vi "Main.vi"() -> ()   [LabVIEW 2025]
doc: "This template is for the Queued Message Handler design pattern.\n\nThe Event Handling Loop generates messages based on user interface actions.\n\nThe Message Handling Loop processes messages generated by the Event Handling Loop, or by other messages. The messages are string values, so new messages can be added easily to the Message Cases case structure in the Message Handling Loop. Each message cluster can also provide an optional value for Message Data, which is a variant that can be converted to whatever message-specific data is required."
uses:
  support/Message Queue/Enqueue Message (Single).vi
  <vilib>/Utility/error.llb/Error Cluster From Error Code.vi
  <vilib>/ErrorRing/Error Ring.xnode
  support/Message Queue/Message Queue.lvlib
  support/User Event - Stop/User Event - Stop.lvlib
panel:
  out "Status":string
  out "Counter Status":bool
  in  "Speed: [Knob: 1-5]":i32(knob) scale=1.0..5.0
  in  "Pause":bool
  in  "Play":bool
  out "Counter":dbl
  in  "Exit":bool
  # "Counter"
  # "Use the Play, Pause, and Exit buttons to control the primary counting function.\n\nThe Play button initiates or resumes the counter.\nPause will temporarily halt the counter, allowing you to resume from the same value. Exit will stop all processes and close the application.\nThe Speed knob allows you to adjust how quickly the counter increments, with higher numbers typically representing faster counting.\n\nThe current count is always visible in the Counter display. The counter will stop if it hits the threshold value. You can adjust this threshold value in the block diagram."
  # "(1=Slow, 5=Fast)"
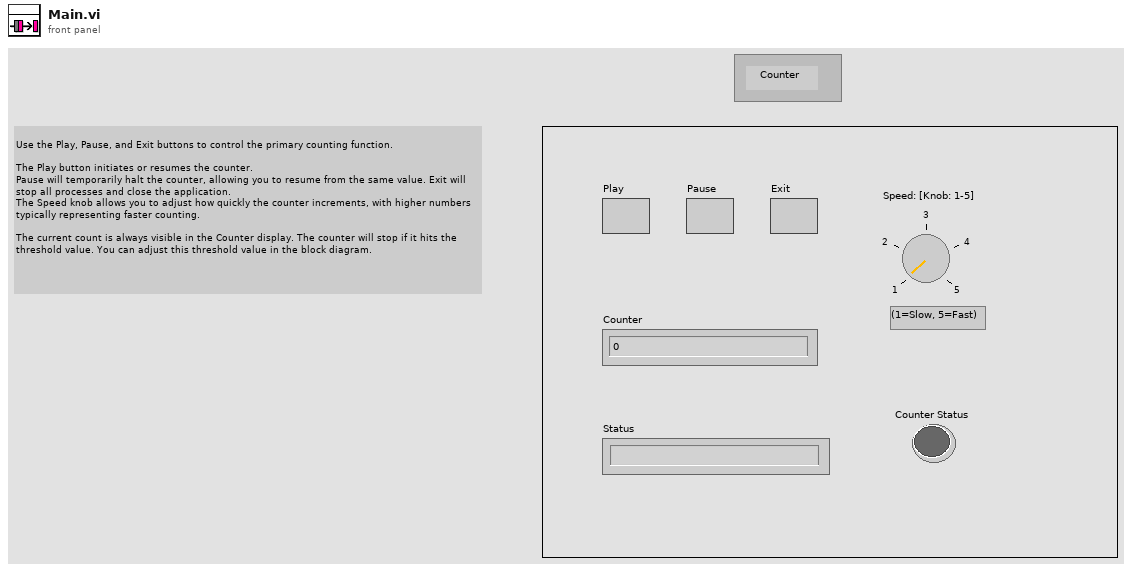
[diagram p1: front panel]
types:
  T1 = cluster{"Boolean <Replace Me>":bool, "String <Replace Me>":string, "Counter":dbl, "is Running":bool, "speed":dbl}
  T2 = typedef "Message Queue.lvlib/All Message Queues.ctl" = cluster{"UI":refnum<queue>}
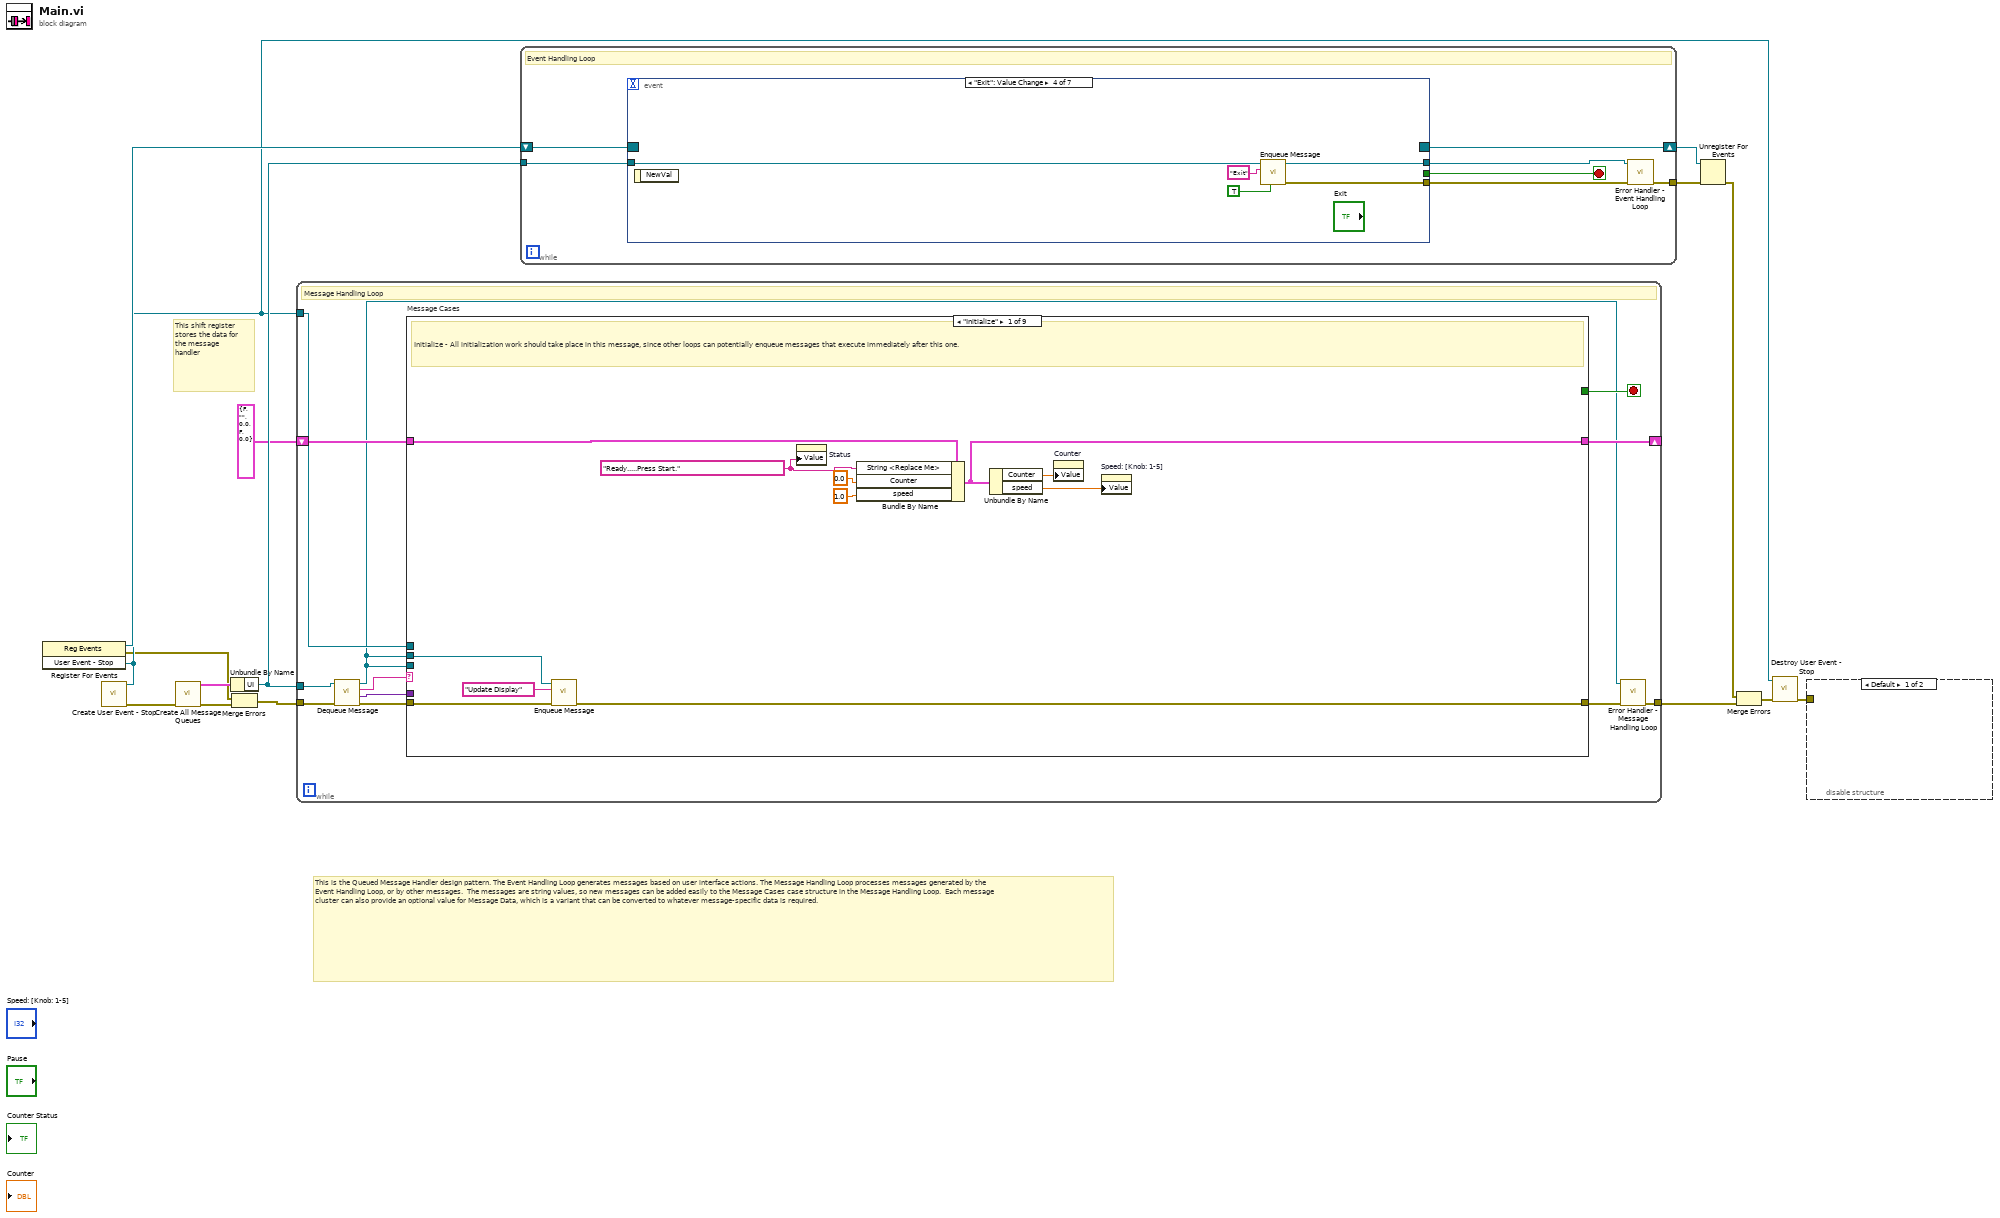
[diagram p0: block diagram]
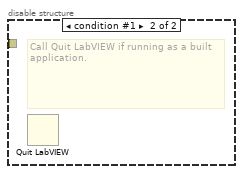
[diagram p2: hidden frame]
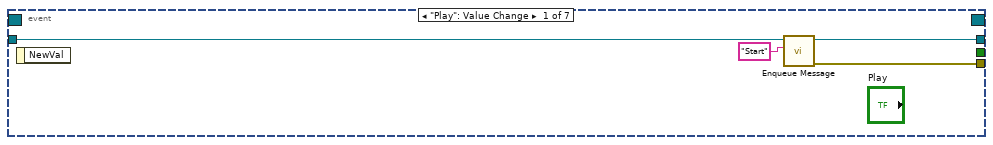
[diagram p3: hidden frame]
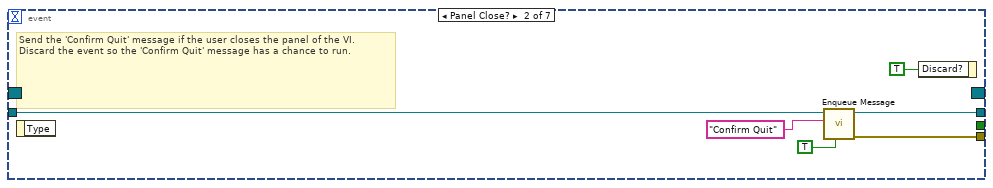
[diagram p4: hidden frame]
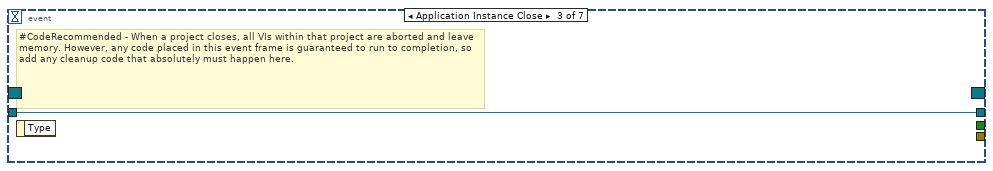
[diagram p5: hidden frame]
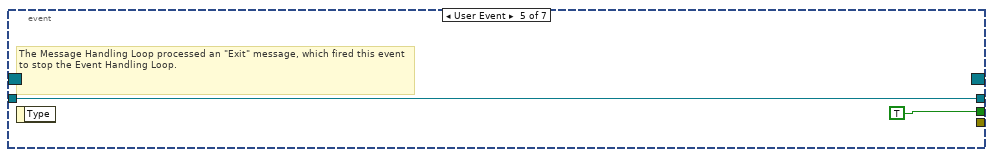
[diagram p6: hidden frame]
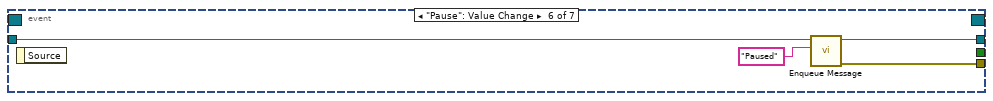
[diagram p7: hidden frame]
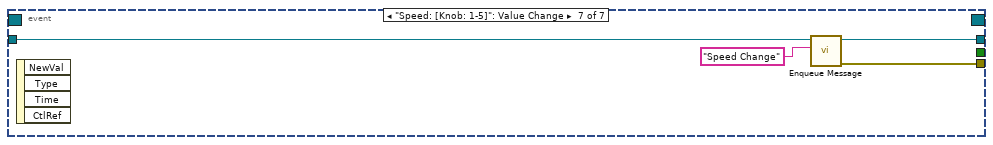
[diagram p8: hidden frame]
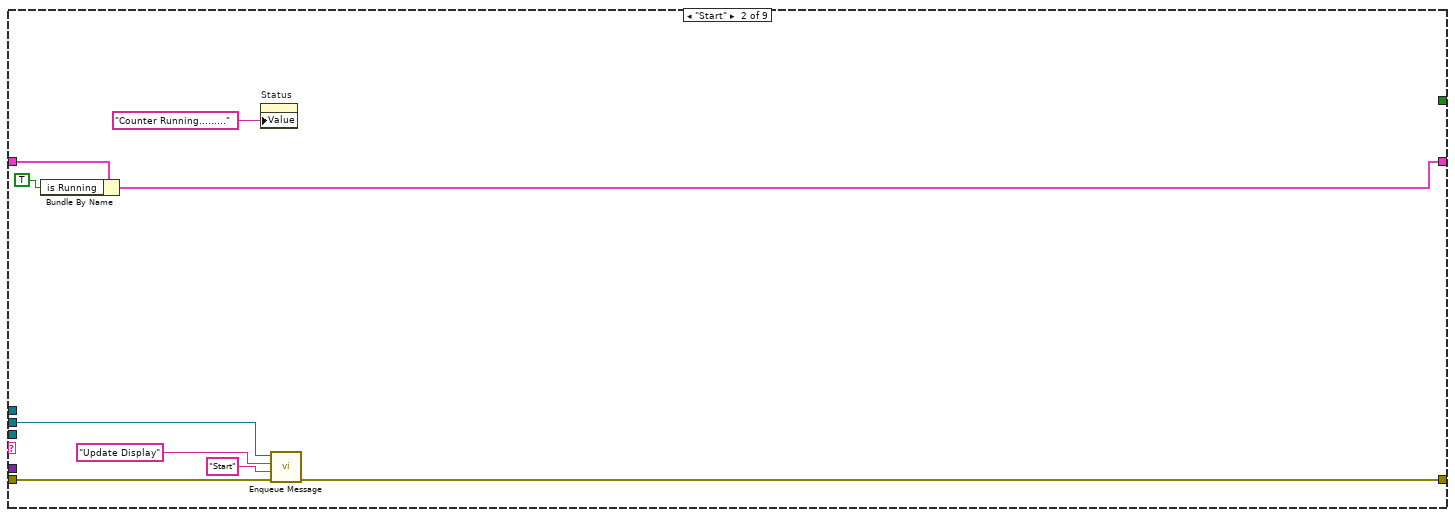
[diagram p9: hidden frame]
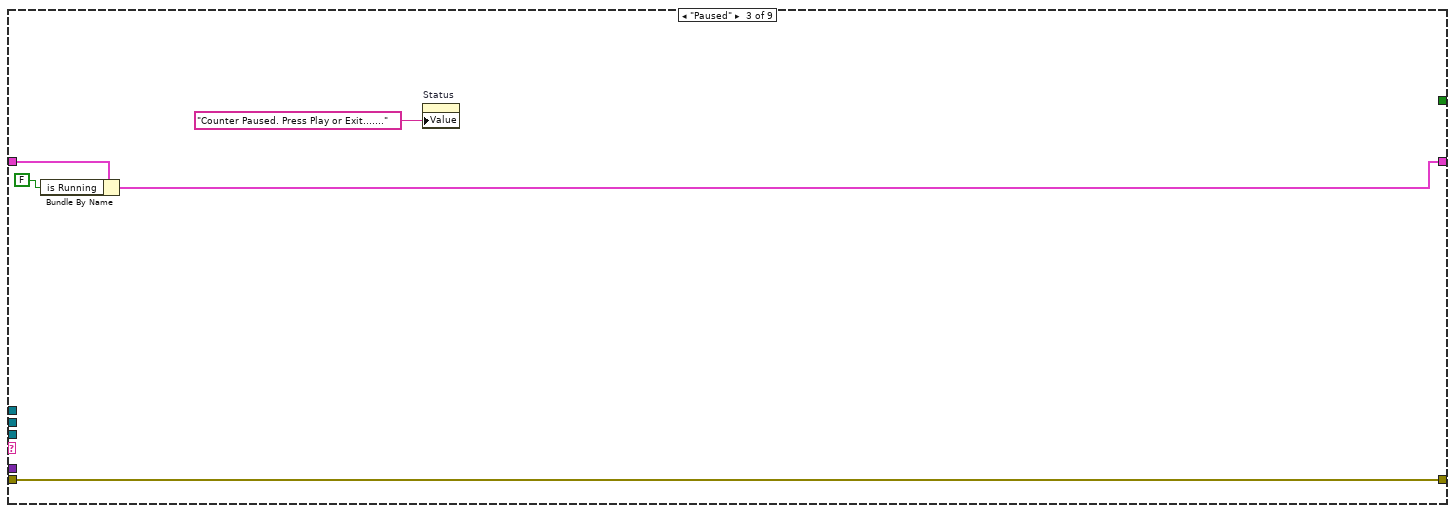
[diagram p10: hidden frame]
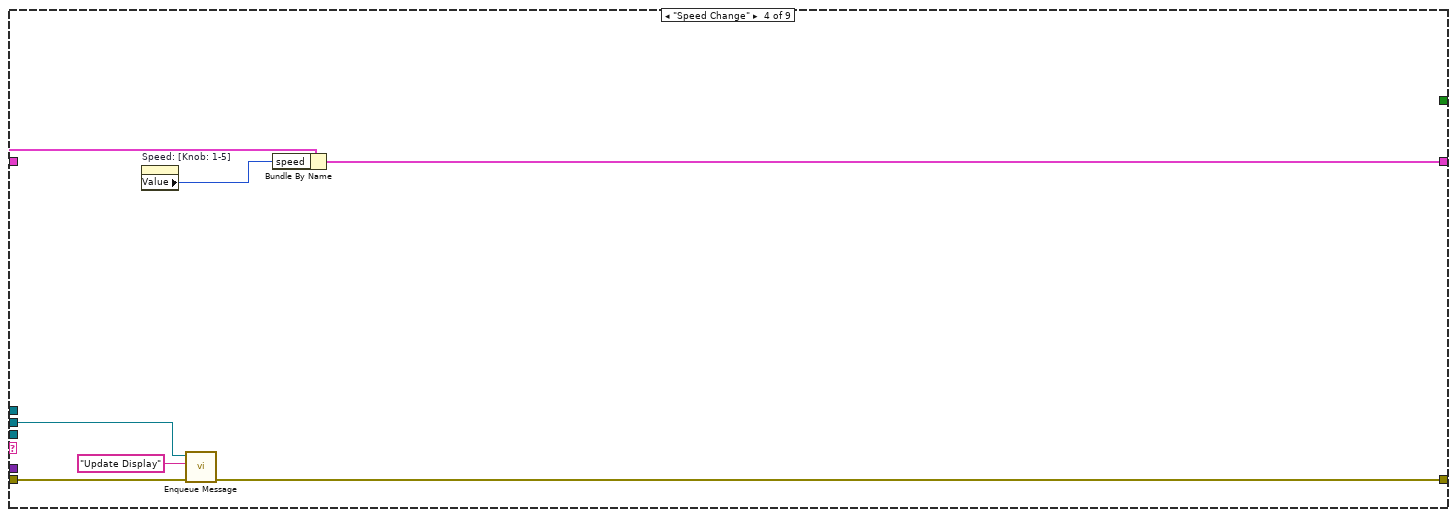
[diagram p11: hidden frame]
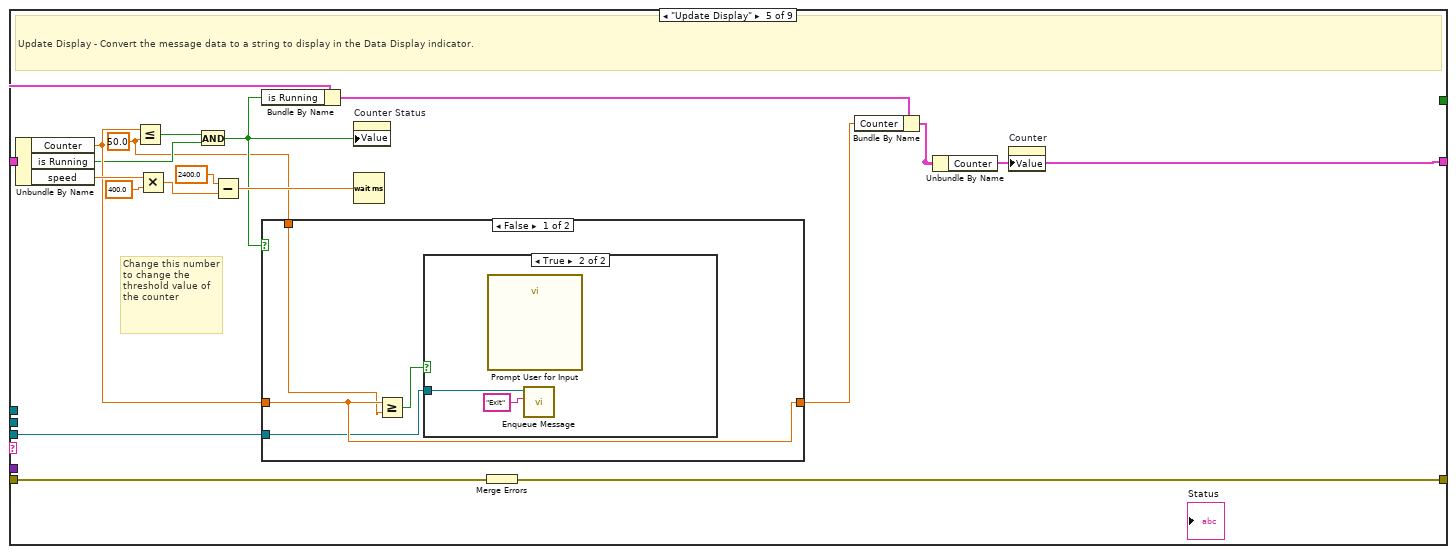
[diagram p12: hidden frame]
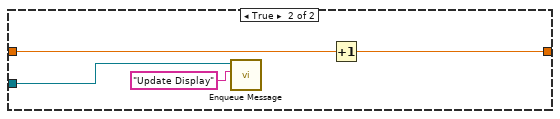
[diagram p14: hidden frame]
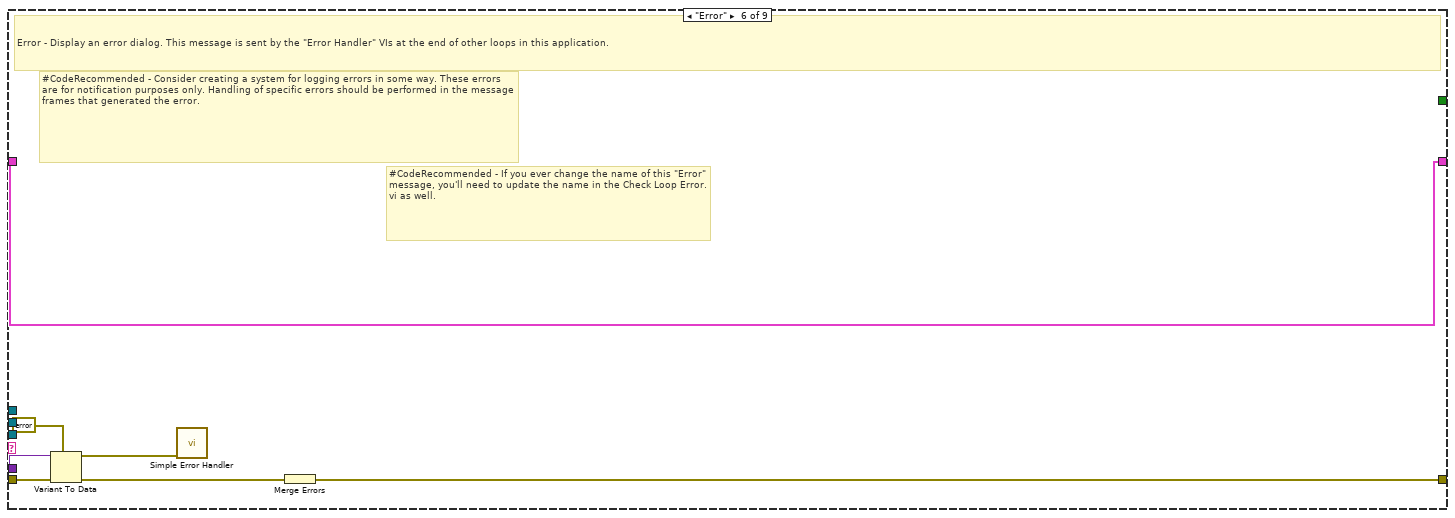
[diagram p15: hidden frame]
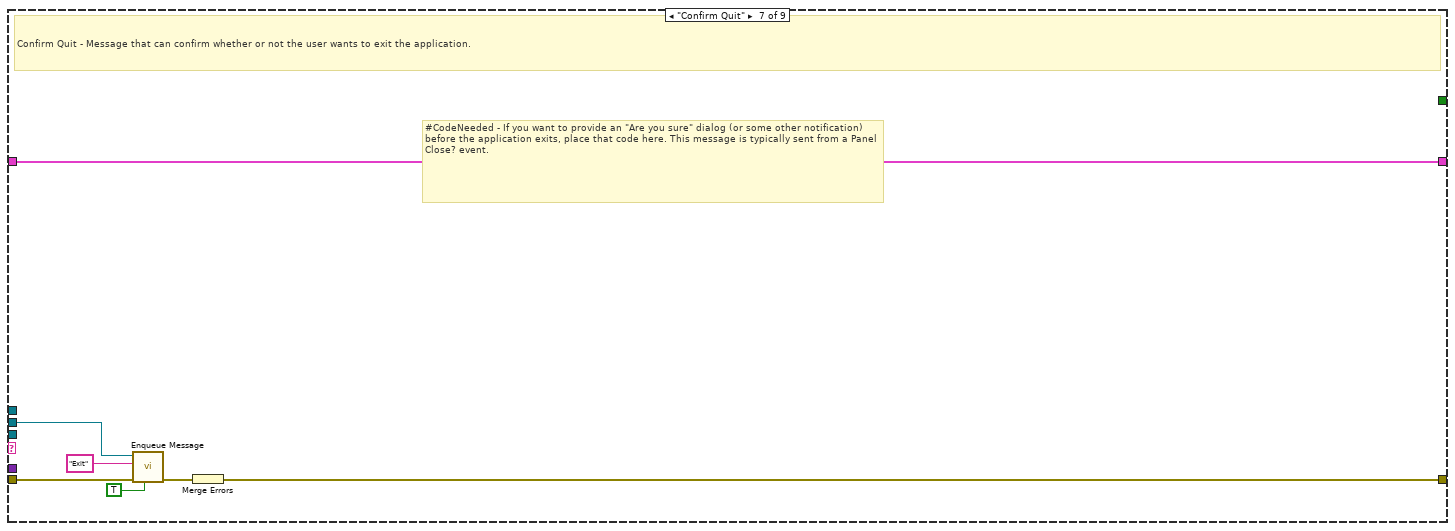
[diagram p16: hidden frame]
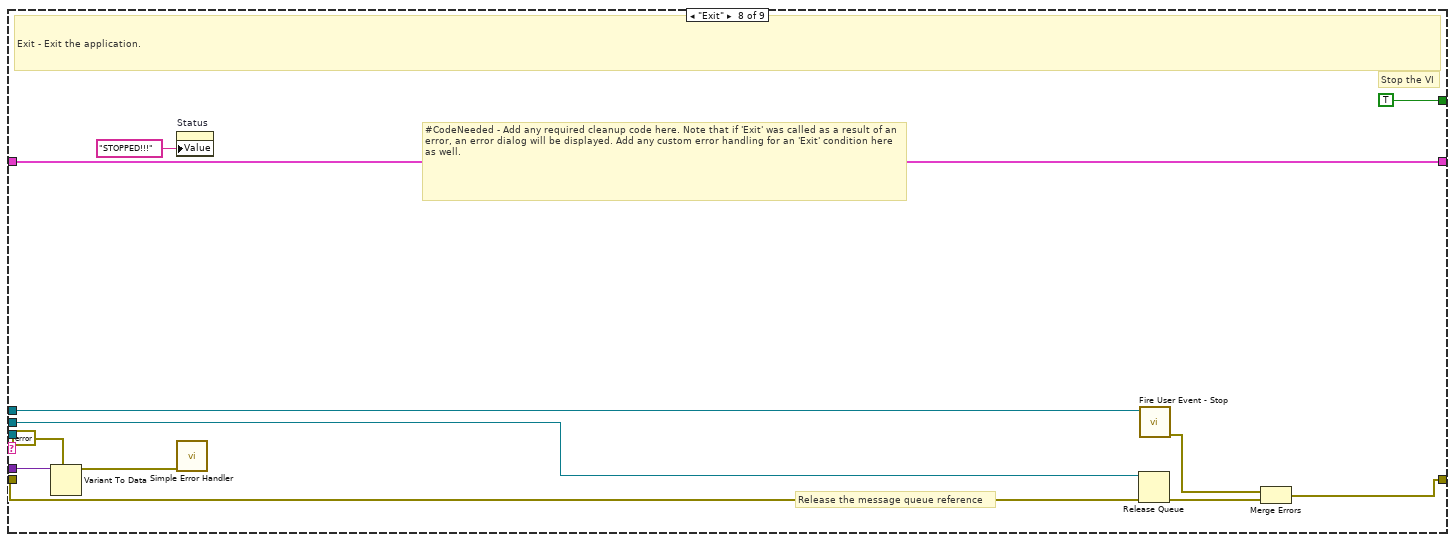
[diagram p17: hidden frame]
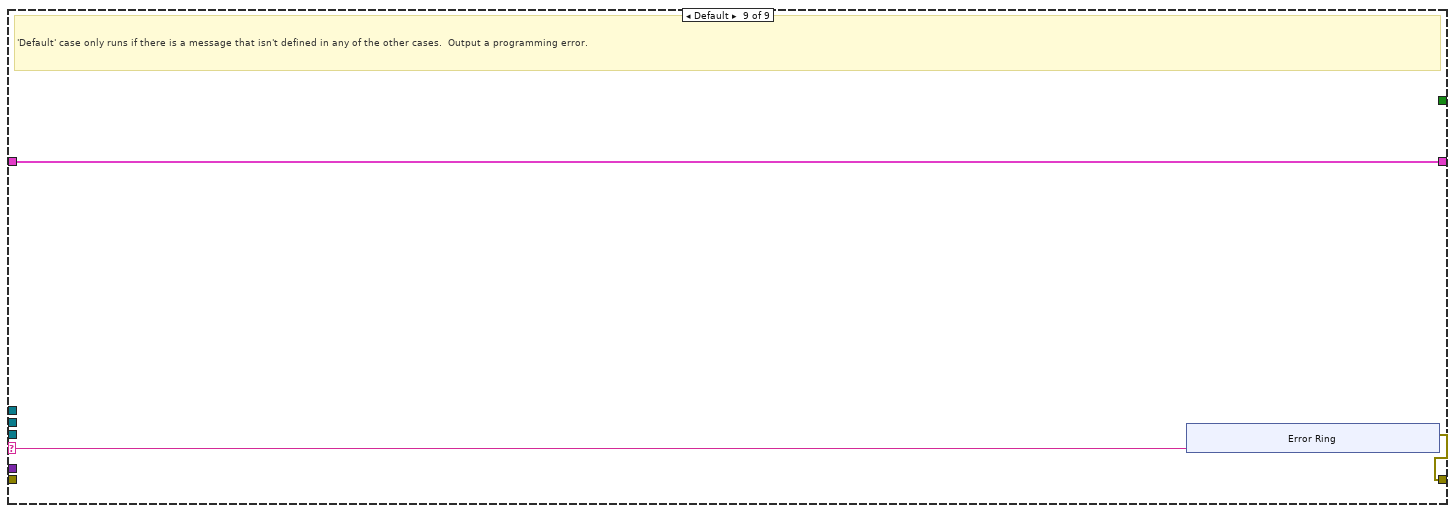
[diagram p18: hidden frame]
diagram:
  # "This is the Queued Message Handler design pattern. The Event Handling Loop generates messages based on user interface actions. The Message Handling Loop processes messages generated by the Event Handling Loop, or by other messages.  The messages are string values, so new messages can be added easily to the Message Cases case structure in the Message Handling Loop.  Each message cluster can also provide an optional value for Message Data, which is a variant that can be converted to whatever message-specific data is required."
  # "This shift register stores the data for the message handler"
  n1 = call "Create User Event - Stop.vi"() -> ("error out"=w11:errorcluster, "User Event - Stop"=w4:refnum<user-event>)  [unwired: 10 in]
  n2 = register-events(w4) -> (reference out=w5:refnum<event-registration>, error out=w2:errorcluster)  [unwired: 2 in]
  n3 = call "Create All Message Queues.vi"("error in (no error)"=w11) -> ("error out"=w15:errorcluster, "Message Queues out"=w14:T2)  [unwired: 9 in]
  n4 = Unbundle By Name(w14) -> ("UI"=w12:refnum<queue>)
  n5 = Merge Errors(w2, w15) -> (w3:errorcluster)
  n6 = while {
    tunnel: w12 -> [w20]
    shift-right: [w17] -> _
    shift-left: T1 {"Boolean <Replace Me>"=FALSE, "String <Replace Me>"="", "Counter"=0.0, "is Running"=FALSE, "speed"=0.0} ("UI Data") -> [w27]
    tunnel: w4 -> [w25]
    tunnel: w3 -> [w24]
    tunnel: [w19] -> w13
    stop <- w26 stop-if-true
    # "Message Handling Loop"
    n7 = call "Dequeue Message.vi"("error in (no error)"=w24, "Message Queue"=w20) -> ("error out"=w23:errorcluster, "Message Data"=w21:variant, "Message"=w22:string, "dup Message Queue"=w16:refnum<queue>)  [unwired: 6 in]
    n8 = case "Message Cases" shown="\"Initialize\"" w22 {
      selector: w22 -> [_ _ _ _ _ _ _ _ w114]
      tunnel: w16 -> [w35 w47 _ w57 _ _ w97 w113 _]
      tunnel: w23 -> [w37 w44 w52 w56 w68 w94 w101 w106 _]
      tunnel: [w38 w43 w52 w58 w67 w88 w99 w109 w115] -> w18
      tunnel: w27 -> [w34 w42 w51 w55 w63 w93 w100 w112 w116]
      tunnel: [w32 w40 w50 w53 w76 w93 w100 w112 w116] -> w17
      tunnel: [_ _ _ _ _ _ _ TRUE _] -> w26
      tunnel: w21 -> [_ _ _ _ _ w92 _ w103 _]
      tunnel: w25 -> [_ _ _ _ _ _ _ w108 _]
      tunnel: w16 -> [_ _ _ _ w74 _ _ _ _]
      frame "Initialize" {
        w28 = "Ready.....Press Start." ("Initial Message")
        # "Initialize - All initialization work should take place in this message, since other loops can potentially enqueue messages that execute immediately after this one."
        n9 = call-poly "Enqueue Message.vi"("error in (no error)"=w37, "Message"="Update Display", "Message Queue"=w35) -> ("error out"=w38:errorcluster)  [unwired: 7 in, 1 out]
        n10 = property on="Status" class="Str"("Value"=w28) -> ()  [unwired: 2 in, 2 out]
        n11 = Bundle By Name(cluster=w34, "String <Replace Me>"=w28, "Counter"=0.0 ("Numeric <Replace Me>"), "speed"=1.0) -> (w32:T1)
        n12 = Unbundle By Name(w32) -> ("Counter"=w31:dbl, "speed"=w29:dbl)
        n13 = property on="Counter" class="DigNum (strict)"("Value"=w31) -> ()  [unwired: 2 in, 2 out]
        n14 = property on="Speed: [Knob: 1-5]" class="Knob (strict)"("Value"=w29) -> ()  [unwired: 2 in, 2 out]
      }
      frame "Start" {
        n15 = Bundle By Name(cluster=w42, "is Running"=TRUE) -> (w40:T1)
        n16 = property on="Status" class="Str"("Value"="Counter Running.........") -> ()  [unwired: 2 in, 2 out]
        n17 = call-poly "Enqueue Message.vi"("error in (no error)"=w44, "Message Data"="Start", "Message"="Update Display", "Message Queue"=w47) -> ("error out"=w43:errorcluster)  [unwired: 6 in, 1 out]
      }
      frame "Paused" {
        n18 = Bundle By Name(cluster=w51, "is Running"=FALSE) -> (w50:T1)
        n19 = property on="Status" class="Str"("Value"="Counter Paused. Press Play or Exit.......") -> ()  [unwired: 2 in, 2 out]
      }
      frame "Speed Change" {
        n20 = property on="Speed: [Knob: 1-5]" class="Knob (strict)"() -> ("Value"=w54:i32)  [unwired: 2 in, 2 out]
        n21 = call-poly "Enqueue Message.vi"("error in (no error)"=w56, "Message"="Update Display", "Message Queue"=w57) -> ("error out"=w58:errorcluster)  [unwired: 7 in, 1 out]
        n22 = Bundle By Name(cluster=w55, "speed"=w54) -> (w53:T1)
      }
      frame "Update Display" {
        w60 = 50.0 ("y")
        # "Change this number to change the threshold value of the counter"
        # "Update Display - Convert the message data to a string to display in the Data Display indicator."
        n23 = Unbundle By Name(w63) -> ("Counter"=w66:dbl, "is Running"=w64:bool, "speed"=w73:dbl)
        n24 = Less Or Equal?(x=w66, y=w60) -> (x <= y?=w65:bool)
        n25 = Multiply(x=w73, y=400.0) -> (x*y=w71:dbl)
        n26 = And(x=w65, y=w64) -> (x .and. y?=w61:bool)
        n27 = Subtract(x=2400.0, y=w71) -> (x-y=w69:dbl)
        n28 = Bundle By Name(cluster=w63, "is Running"=w61) -> (w62:T1)
        n29 = case shown="False" w61 {
          tunnel: w66 -> [w81 w87]
          tunnel: [w81 w86] -> w77
          tunnel: w74 -> [w79 w85]
          tunnel: w60 -> [w78 _]
          frame False {
            n30 = Greater Or Equal?(x=w81, y=w78) -> (x >= y?=w80:bool)
            n31 = case shown="True" w80 {
              tunnel: w79 -> [_ w83]
              frame False {
              }
              frame True {
                n32 = call "Prompt User for Input"() -> ()  [unwired: 18 in, 2 out]
                n33 = call-poly "Enqueue Message.vi"("Message"="Exit", "Message Queue"=w83) -> ()  [unwired: 8 in, 2 out]
              }
            }
          }
          frame True {
            n34 = call-poly "Enqueue Message.vi"("Message"="Update Display", "Message Queue"=w85) -> ()  [unwired: 8 in, 2 out]
            n35 = Increment(x=w87) -> (x+1=w86:dbl)
          }
        }
        n36 = property on="Counter Status" class="Bool (strict)"("Value"=w61) -> ()  [unwired: 2 in, 2 out]
        n37 = Wait (ms)(milliseconds to wait=w69) -> ()  [unwired: 1 out]
        n38 = Merge Errors(w68) -> (w67:errorcluster)
        n39 = Bundle By Name(cluster=w62, "Counter"=w77) -> (w76:T1)
        n40 = Unbundle By Name(w76) -> ("Counter"=w75:dbl)
        n41 = property on="Counter" class="DigNum (strict)"("Value"=w75) -> ()  [unwired: 2 in, 2 out]
      }
      frame "Error" {
        # "#CodeRecommended - If you ever change the name of this \"Error\" message, you'll need to update the name in the Check Loop Error.vi as well."
        # "#CodeRecommended - Consider creating a system for logging errors in some way. These errors are for notification purposes only. Handling of specific errors should be performed in the message frames that generated the error."
        # "Error - Display an error dialog. This message is sent by the \"Error Handler\" VIs at the end of other loops in this application."
        n42 = Variant To Data(error in=w94, type=errorcluster {"status"=FALSE, "code"=0, "source"=""} ("error constant"), Variant=w92) -> (data=w90:errorcluster, error out=w89:errorcluster)
        n43 = call <vilib>:"Simple Error Handler.vi"("error in (no error)"=w90) -> ()  [unwired: 4 in, 5 out]
        n44 = Merge Errors(w89) -> (w88:errorcluster)
      }
      frame "Confirm Quit" {
        # "#CodeNeeded - If you want to provide an \"Are you sure\" dialog (or some other notification) before the application exits, place that code here. This message is typically sent from a Panel Close? event."
        # "Confirm Quit - Message that can confirm whether or not the user wants to exit the application."
        n45 = call-poly "Enqueue Message.vi"("Priority Message? (F)"=TRUE, "error in (no error)"=w101, "Message"="Exit", "Message Queue"=w97) -> ("error out"=w98:errorcluster)  [unwired: 6 in, 1 out]
        n46 = Merge Errors(w98) -> (w99:errorcluster)
      }
      frame "Exit" {
        # "Stop the VI"
        # "Release the message queue reference"
        # "#CodeNeeded - Add any required cleanup code here. Note that if 'Exit' was called as a result of an error, an error dialog will be displayed. Add any custom error handling for an 'Exit' condition here as well."
        # "Exit - Exit the application."
        n47 = Variant To Data(type=errorcluster {"status"=FALSE, "code"=0, "source"=""} ("error constant"), Variant=w103) -> (data=w104:errorcluster)  [unwired: 1 in, 1 out]
        n48 = property on="Status" class="Str"("Value"="STOPPED!!!") -> ()  [unwired: 2 in, 2 out]
        n49 = call <vilib>:"Simple Error Handler.vi"("error in (no error)"=w104) -> ()  [unwired: 4 in, 5 out]
        n50 = Release Queue(queue=w113, error in (no error)=w106) -> (error out=w110:errorcluster)  [unwired: 1 in, 2 out]
        n51 = call "Fire User Event - Stop.vi"("User Event - Stop"=w108) -> ("error out"=w107:errorcluster)  [unwired: 10 in]
        n52 = Merge Errors(w107, w110) -> (w109:errorcluster)
      }
      frame Default {
        # "'Default' case only runs if there is a message that isn't defined in any of the other cases.  Output a programming error."
        n53 = xnode "Error Ring"("parameter 0"=w114) -> ("error out"=w115:errorcluster)
      }
    }
    n54 = call "Error Handler - Message Handling Loop.vi"("error in (no error)"=w18, "Message Queue"=w16) -> ("dup error in"=w19:errorcluster)  [unwired: 8 in, 1 out]
  }
  n55 = while {
    tunnel: w12 -> [w130]
    shift-right: [w128] -> w8
    shift-left: w5 -> [w129]
    tunnel: [w124] -> w6
    stop <- w126 stop-if-true
    # "Event Handling Loop"
    n56 = event shown="[3] \"Exit\": Value Change" {
      selector: w129 -> [_ _ _ _ _ _ _]
      dyn-events: [_ _ _ _ _ _ _] -> w128
      timeout: _ -> [_ _ _ _ _ _ _]
      tunnel: [_ _ _ _ TRUE ("Discard?") _ _] -> w126
      tunnel: w130 -> [w133 w139 w141 w146 w148 w151 w156]
      tunnel: [w131 w138 _ w145 _ w150 w153] -> w127
      tunnel: [w132 w137 w141 w144 w148 w149 w155] -> w125
      event "Play": Value Change {
        n57 = event-data() -> ()  [unwired: 1 in, 1 out]
        n58 = call-poly "Enqueue Message.vi"("Message"="Start", "Message Queue"=w133) -> ("error out"=w131:errorcluster, "dup Message Queue"=w132:refnum<queue>)  [unwired: 8 in]
      }
      event Panel Close? {
        # "Send the 'Confirm Quit' message if the user closes the panel of the VI. Discard the event so the 'Confirm Quit' message has a chance to run."
        n59 = event-data() -> ()  [unwired: 1 in, 1 out]
        n60 = call-poly "Enqueue Message.vi"("Priority Message? (F)"=TRUE, "Message"="Confirm Quit", "Message Queue"=w139) -> ("error out"=w138:errorcluster, "dup Message Queue"=w137:refnum<queue>)  [unwired: 7 in]
        n61 = event-data("Discard?"=TRUE) -> ()  [unwired: 1 in, 1 out]
      }
      event Application Instance Close {
        # "#CodeRecommended - When a project closes, all VIs within that project are aborted and leave memory. However, any code placed in this event frame is guaranteed to run to completion, so add any cleanup code that absolutely must happen here."
        n62 = event-data() -> ()  [unwired: 1 in, 1 out]
      }
      event "Exit": Value Change {
        n63 = event-data() -> ()  [unwired: 1 in, 1 out]
        n64 = call-poly "Enqueue Message.vi"("Priority Message? (F)"=TRUE, "Message"="Exit", "Message Queue"=w146) -> ("error out"=w145:errorcluster, "dup Message Queue"=w144:refnum<queue>)  [unwired: 7 in]
      }
      event User Event {
        # "The Message Handling Loop processed an \"Exit\" message, which fired this event to stop the Event Handling Loop."
        n65 = event-data() -> ()  [unwired: 1 in, 1 out]
      }
      event "Pause": Value Change {
        n66 = event-data() -> ()  [unwired: 1 in, 1 out]
        n67 = call-poly "Enqueue Message.vi"("Message"="Paused", "Message Queue"=w151) -> ("error out"=w150:errorcluster, "dup Message Queue"=w149:refnum<queue>)  [unwired: 8 in]
      }
      event "Speed: [Knob: 1-5]": Value Change {
        n68 = event-data() -> ()  [unwired: 1 in, 4 out]
        n69 = call-poly "Enqueue Message.vi"("Message"="Speed Change", "Message Queue"=w156) -> ("error out"=w153:errorcluster, "dup Message Queue"=w155:refnum<queue>)  [unwired: 8 in]
      }
    }
    n70 = call "Error Handler - Event Handling Loop.vi"("error in (no error)"=w127, "Message Queue"=w125) -> ("dup error in"=w124:errorcluster)  [unwired: 8 in, 1 out]
  }
  n71 = Unregister For Events(event registration refnum=w8, error in=w6) -> (error out=w9:errorcluster)
  n72 = Merge Errors(w9, w13) -> (w10:errorcluster)
  n73 = call "Destroy User Event - Stop.vi"("error in (no error)"=w10, "User Event - Stop"=w4) -> ("error out"=w7:errorcluster)  [unwired: 9 in]
  n74 = disable-structure shown="Default" {
    disable-tunnel: w7 -> [_ _]
    frame condition #0 (active) {
    }
    frame condition #1 {
      # "Call Quit LabVIEW if running as a built application."
      n75 = Quit LabVIEW() -> ()  [unwired: 1 in]
    }
  }
